vi "Stop Task.vi"(8 "error in":errorcluster, 11 "NI PWM Output in":refnum<class "NI PWM Output.lvclass">) -> (0 "error out":errorcluster, 3 "NI PWM Output out":refnum<class "NI PWM Output.lvclass">)   [LabVIEW 2023, in "HardwareAbstractionLayer_LVOOP.lvlib" / "NI PWM Output.lvclass"]
doc: "This VI is DAQmx Stop the Task"
uses:
  NI PWM Output.lvclass
  NI PWM Output.lvclass/NI PWM Output.ctl
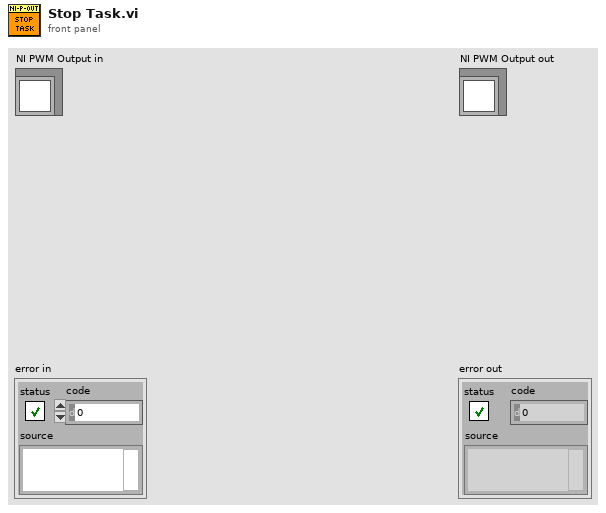
[diagram p1: front panel]
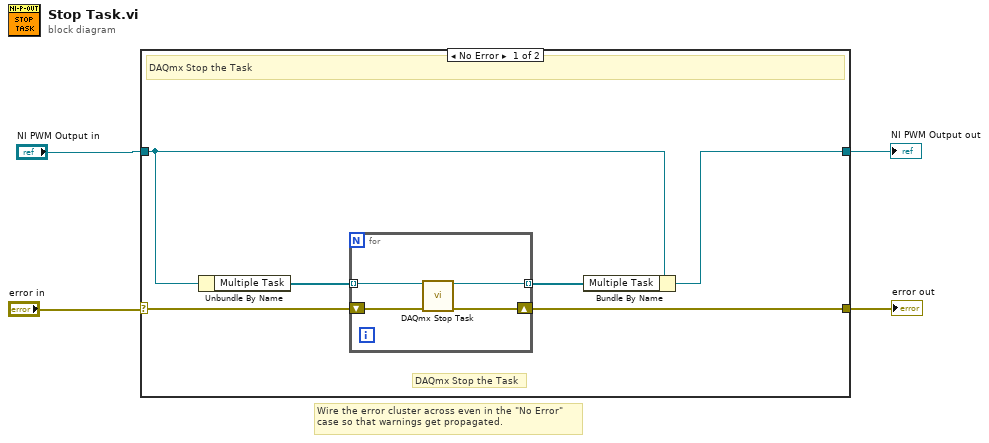
[diagram p0: block diagram]
diagram:
  # "Wire the error cluster across even in the \"No Error\"\ncase so that warnings get propagated."
  n1 = case shown="No Error" "error in" {
    selector: "error in" -> [w10 w16]
    tunnel: [w9 w16] -> w3
    tunnel: [w6 w15] -> w1
    tunnel: "NI PWM Output in" -> [w7 w15]
    frame No Error {
      # "DAQmx Stop the Task"
      # "DAQmx Stop the Task"
      n2 = Unbundle By Name(w7) -> ("Multiple Task"=w8:refnum<k21>[])
      n3 = for {
        tunnel: w8 -> [w13] mode=indexing
        shift-right: [w12] -> w9
        shift-left: w10 -> [w14]
        tunnel: [w11] -> w5 mode=indexing
        n4 = call <vilib>:"DAQmx Stop Task.vi"("task/channels in"=w13, "error in"=w14) -> ("task out"=w11:refnum<k21>, "error out"=w12:errorcluster)  [unwired: 12 in]
      }
      n5 = Bundle By Name(cluster=w7, "Multiple Task"=w5) -> (w6:refnum<class "NI PWM Output.lvclass">)
    }
    frame Error {
    }
  }
  "error out" <- w3
  "NI PWM Output out" <- w1
